vi "RESET.vi"(8 "Error":errorcluster, 11 "FP":refnum<class "DecFrame_FP.lvclass">) -> (0 "Error Out":errorcluster, 3 "FP Out":refnum<class "DecFrame_FP.lvclass">)   [LabVIEW 2025, in "DecFrame_FP.lvclass"]
uses:
  DecFrame_FP.lvclass
  TypeDefs_Utility/Cluster_FP_Scroll Bars Hide Show.ctl
  TypeDefs_Utility/ENUM_FP_Show-Hide Select.ctl
  TypeDefs_Utility/Cluster_FP_Show Hide Items.ctl
  DecFrame_FP.lvclass/DecFrame_FP.ctl
  FPEN/FPEN.lvclass
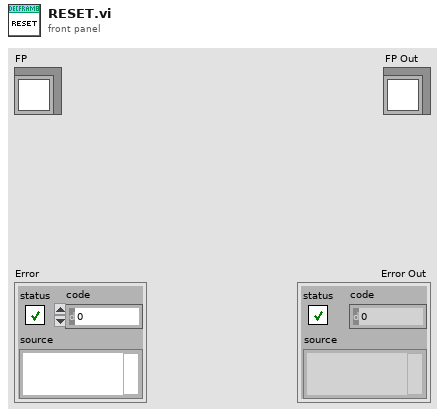
[diagram p1: front panel]
types:
  T1 = typedef "Cluster_FP_Show Hide Items.ctl" = cluster{"MenuBar":T2, "FreeRunButton":T2, "RunButton":T2, "AbortButton":T2, "ToolBar":T2, "Resize":T2, "Closeable":T2, "Minimizable":T2}
  T2 = typedef "ENUM_FP_Show-Hide Select.ctl" = enum16{"No Change", "Hide", "Show"}
  T3 = typedef "Cluster_FP_Scroll Bars Hide Show.ctl" = cluster{"Horiz SBar":T2, "Vert SBar":T2}
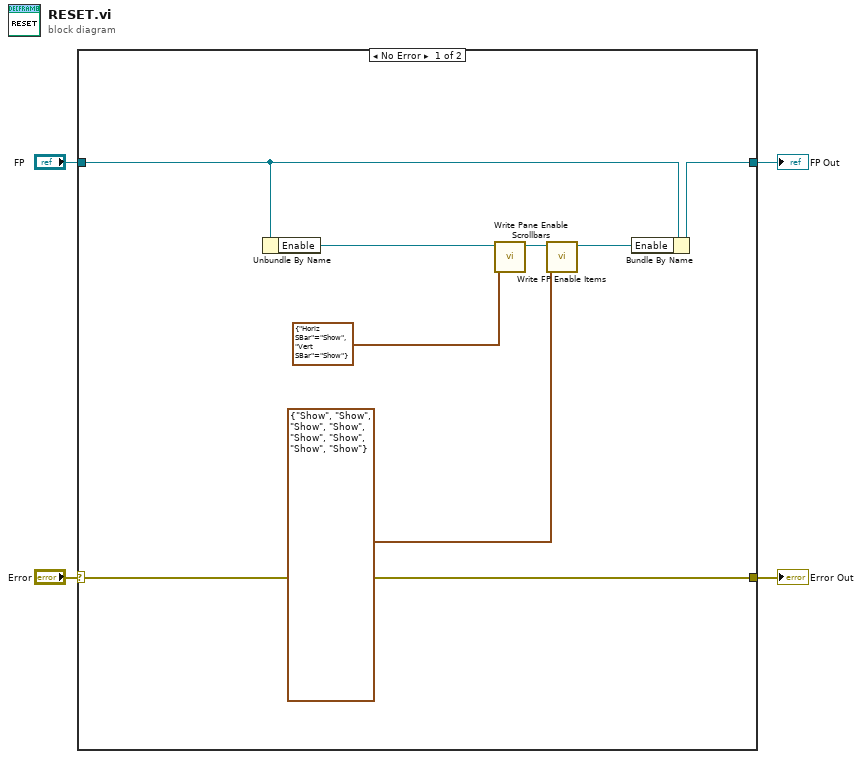
[diagram p0: block diagram]
diagram:
  n1 = case shown="No Error" "Error" {
    selector: "Error" -> [w5 w14]
    tunnel: [w5 w14] -> w3
    tunnel: [w11 w13] -> w1
    tunnel: "FP" -> [w12 w13]
    frame No Error {
      n2 = Unbundle By Name(w12) -> ("Enable"=w7:refnum<class "FPEN.lvclass">)
      n3 = call "Write Pane Enable Scrollbars.vi"("Pane"=T3 {"Horiz SBar"=enum."Show", "Vert SBar"=enum."Show"} ("Scrollbar Settings"), "FPEN"=w7) -> ("FPEN Out"=w8:refnum<class "FPEN.lvclass">)  [unwired: 9 in]
      n4 = call "Write FP Enable Items.vi"("FP Enable Items"=T1 {"MenuBar"=enum."Show", "FreeRunButton"=enum."Show", "RunButton"=enum."Show", "AbortButton"=enum."Show", "ToolBar"=enum."Show", "Resize"=enum."Show", "Closeable"=enum."Show", "Minimizable"=enum."Show"} ("FP Show Hide"), "FPEN"=w8) -> ("FPEN Out"=w6:refnum<class "FPEN.lvclass">)  [unwired: 9 in]
      n5 = Bundle By Name(cluster=w12, "Enable"=w6) -> (w11:refnum<class "DecFrame_FP.lvclass">)
    }
    frame Error {
    }
  }
  "Error Out" <- w3
  "FP Out" <- w1
